vi "PassKickerRole.vi"(6 "Tactic index in":i32, 7 "first call":bool, 8 "error in (no error)":errorcluster, 10 "Game in":refnum<class "Game.lvclass">, 11 "PassKickerRole in":refnum<class "PassKickerRole.lvclass">) -> (0 "error out":errorcluster, 1 "tactic index":i32, 2 "Robot out":refnum<class "Robot.lvclass">, 3 "PassKickerRole out":refnum<class "PassKickerRole.lvclass">)   [LabVIEW 2023, in "PassKickerRole.lvclass"]
uses:
  PassKickerRole.lvclass
  Robot_class/Robot.lvclass
  Game_class/Game.lvclass
  Role_class/Role.lvclass/Role.ctl
  PassKickerRole.lvclass/PassKickerRole.ctl
  Tacticbook_class/Tacticbook.lvclass/Tacticbook.ctl
  FollowAttackerTactic_class/FollowAttackerTactic.lvclass/FollowAttackerTactic.ctl
  Tacticbook_class/Read FollowAttackerTactic.vi
  FollowAttackerTactic_class/Read States.vi
  Tacticbook_class/Write FollowAttackerTactic.vi
  Role_class/Read Tacticbook.vi
  Read number_of_tactics.vi
  Role_class/Write Tacticbook.vi
  Role_class/Write tactic_index.vi
  Role_class/Read RobotRef.vi
  Tacticbook_class/Tacticbook.lvclass
  FollowAttackerTactic_class/FollowAttackerTactic.lvclass
  KickToPassReceiverTactic_class/KickToPassReceiverTactic.lvclass
panel:
  out "Game out":refnum<class "Game.lvclass">
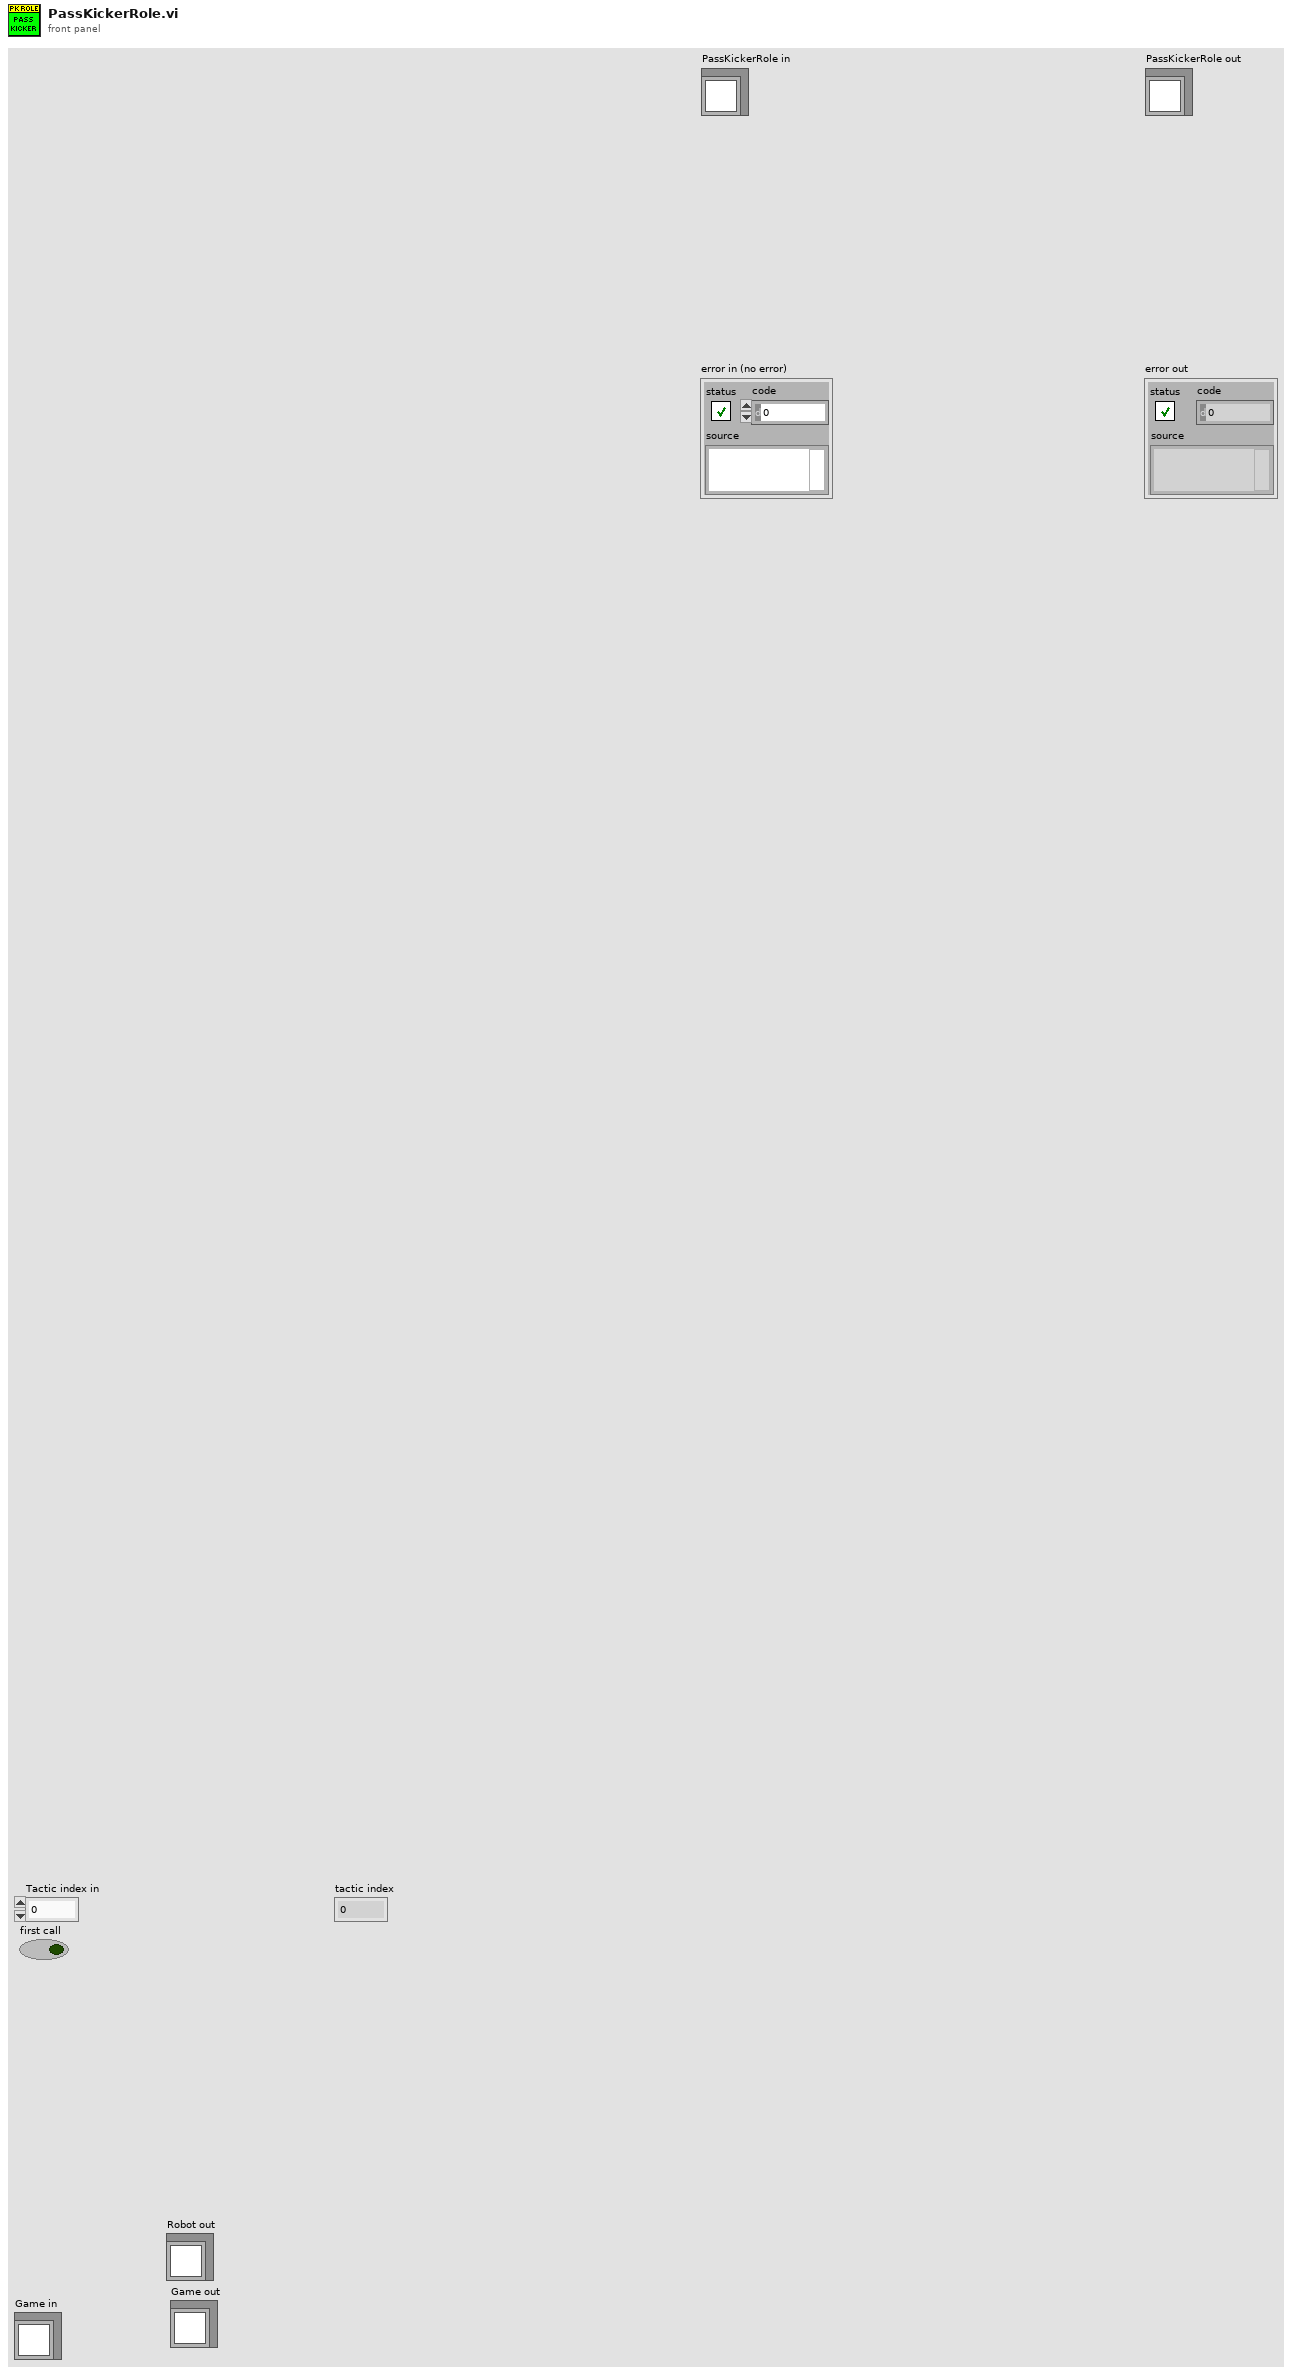
[diagram p1: front panel]
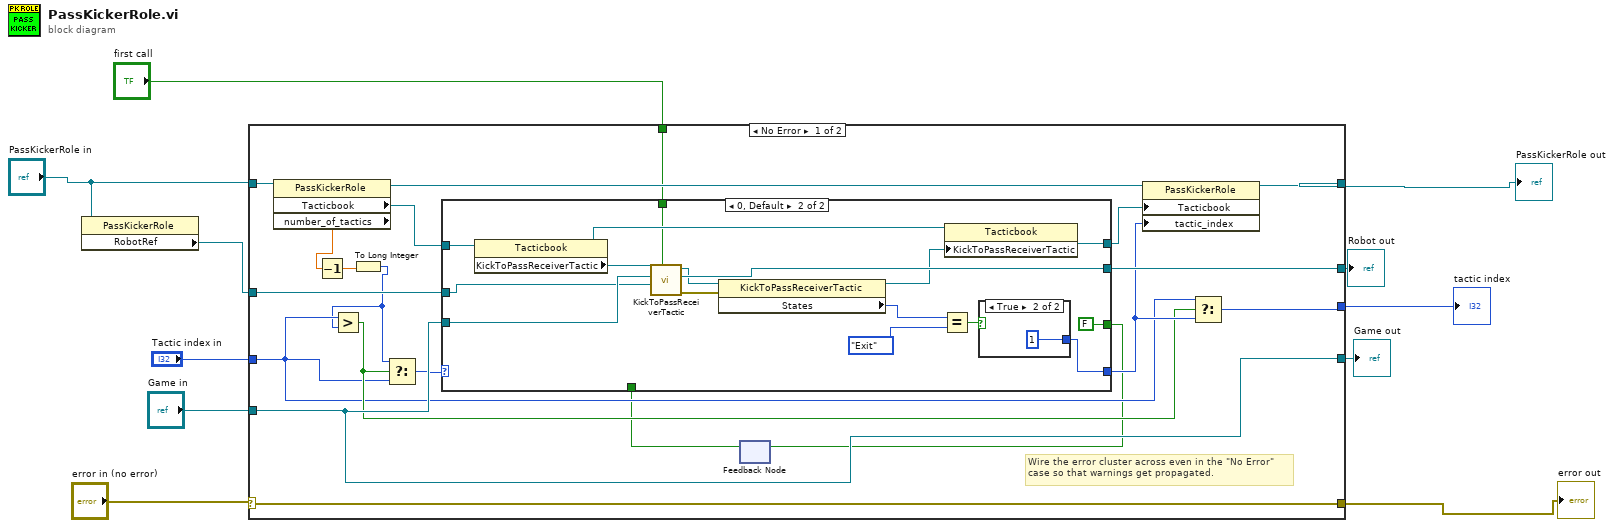
[diagram p0: block diagram]
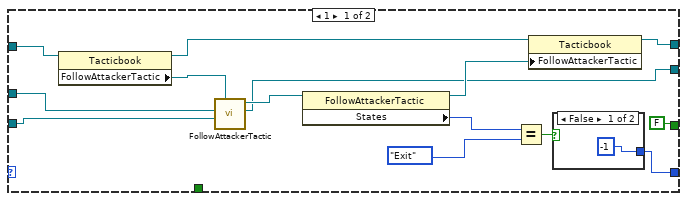
[diagram p2: hidden frame]
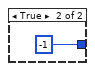
[diagram p3: hidden frame]
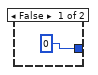
[diagram p4: hidden frame]
diagram:
  n1 = property class="PassKickerRole"(reference="PassKickerRole in") -> ("RobotRef"=w2:refnum<class "Robot.lvclass">)  [unwired: 1 in, 2 out]
  n2 = case shown="No Error" "error in (no error)" {
    selector: "error in (no error)" -> [w31 w69]
    tunnel: [w31 w69] -> w6
    tunnel: [w29 w68] -> w7
    tunnel: "PassKickerRole in" -> [w30 w68]
    tunnel: w2 -> [w26 w67]
    tunnel: [w25 w67] -> w11
    tunnel: [w23 w66] -> w10
    tunnel: "Game in" -> [w23 w66]
    tunnel: [w21 _] -> w5
    tunnel: "Tactic index in" -> [w18 _]
    tunnel: "first call" -> [w16 _]
    frame No Error {
      # "Wire the error cluster across even in the \"No Error\"\ncase so that warnings get propagated."
      n3 = property class="PassKickerRole"(reference=w30) -> (reference out=w28:refnum<class "PassKickerRole.lvclass">, "Tacticbook"=w27:refnum<class "Tacticbook.lvclass">, "number_of_tactics"=w17:dbl)  [unwired: 1 in, 1 out]
      n4 = Decrement(x=w17) -> (x-1=w13:dbl)
      n5 = To Long Integer(number=w13) -> (32bit integer=w12:i32)
      n6 = Greater?(x=w18, y=w12) -> (0:w19:bool)
      n7 = Select(t=w12, s=w19, f=w18) -> (s? t:f=w20:i32)
      n8 = feedback #1() -> (w14:bool)  [unwired: 1 in]
      n9 = case shown="0, Default" w20 {
        tunnel: [w34 w51] -> w22
        tunnel: w27 -> [w43 w63]
        tunnel: w26 -> [w36 w54]
        tunnel: [w37 w62] -> w25
        tunnel: [w41 w58] -> w24
        tunnel: w23 -> [w35 w55]
        tunnel: w16 -> [_ w48]
        tunnel: [FALSE FALSE] -> w15
        tunnel: w14 -> [_ _]
        frame 1 {
          n10 = property class="Tacticbook"(reference=w43) -> (reference out=w42:refnum<class "Tacticbook.lvclass">, "FollowAttackerTactic"=w39:refnum<class "FollowAttackerTactic.lvclass">)  [unwired: 1 in, 1 out]
          n11 = call-dynamic "FollowAttackerTactic.vi"("Game in"=w35, "Robot"=w36, "FollowAttackerTactic in"=w39) -> ("Robot out"=w37:refnum<class "Robot.lvclass">, "FollowAttackerTactic out"=w38:refnum<class "FollowAttackerTactic.lvclass">)  [unwired: 6 in, 1 out]
          n12 = property class="FollowAttackerTactic"(reference=w38) -> (reference out=w40:refnum<class "FollowAttackerTactic.lvclass">, "States"=w44:enum16{"Exit", "FollowAttacker"})  [unwired: 1 in, 1 out]
          n13 = Equal?(x=w44, y=enum16{"Exit", "FollowAttacker"}."Exit" ("States")) -> (x = y?=w45:bool)
          n14 = property class="Tacticbook"(reference=w42, "FollowAttackerTactic"=w40) -> (reference out=w41:refnum<class "Tacticbook.lvclass">)  [unwired: 1 in, 1 out]
          n15 = case shown="False" w45 {
            tunnel: [-1 -1] -> w34
            frame False {
            }
            frame True {
            }
          }
        }
        frame 0, Default {
          n16 = property class="Tacticbook"(reference=w63) -> (reference out=w60:refnum<class "Tacticbook.lvclass">, "KickToPassReceiverTactic"=w57:refnum<class "KickToPassReceiverTactic.lvclass">)  [unwired: 1 in, 1 out]
          n17 = call "KickToPassReceiverTactic.vi"("first call"=w48, "Robot"=w54, "Game in"=w55, "KickToPassReceiverTactic in"=w57) -> ("error out"=w61:errorcluster, "Robot out"=w62:refnum<class "Robot.lvclass">, "KickToPassReceiverTactic out"=w56:refnum<class "KickToPassReceiverTactic.lvclass">)  [unwired: 5 in]
          n18 = property class="KickToPassReceiverTactic"(reference=w56, error in=w61) -> (reference out=w59:refnum<class "KickToPassReceiverTactic.lvclass">, "States"=w52:enum16{"KickToPassReceiver", "WaitPass", "Exit"})  [unwired: 1 out]
          n19 = Equal?(x=w52, y=enum16{"KickToPassReceiver", "WaitPass", "Exit"}."Exit") -> (x = y?=w53:bool)
          n20 = property class="Tacticbook"(reference=w60, "KickToPassReceiverTactic"=w59) -> (reference out=w58:refnum<class "Tacticbook.lvclass">)  [unwired: 1 in, 1 out]
          n21 = case shown="True" w53 {
            tunnel: [0 1] -> w51
            frame False {
            }
            frame True {
            }
          }
        }
      }
      n22 = feedback-in #1(w15) -> ()
      n23 = property class="PassKickerRole"(reference=w28, "Tacticbook"=w24, "tactic_index"=w22) -> (reference out=w29:refnum<class "PassKickerRole.lvclass">)  [unwired: 1 in, 1 out]
      n24 = Select(t=w18, s=w19, f=w22) -> (s? t:f=w21:i32)
    }
    frame Error {
    }
  }
  "error out" <- w6
  "PassKickerRole out" <- w7
  "Robot out" <- w11
  "Game out" <- w10
  "tactic index" <- w5
